vi "getPower.vi"(2 "error in":errorcluster, 3 "AIN Range":u16(ring) items=["LJ_rgBIP10V", "LJ_rgBIP1V", "LJ_rgBIPP1V", "LJ_rgBIPP01V"], 4 "+Channel":u16, 5 "Handle In":i32) -> (0 "error out":errorcluster, 1 "Voltage Reading":dbl)   [LabVIEW 2021]
panel:
  # "inputs"
  # "outputs"
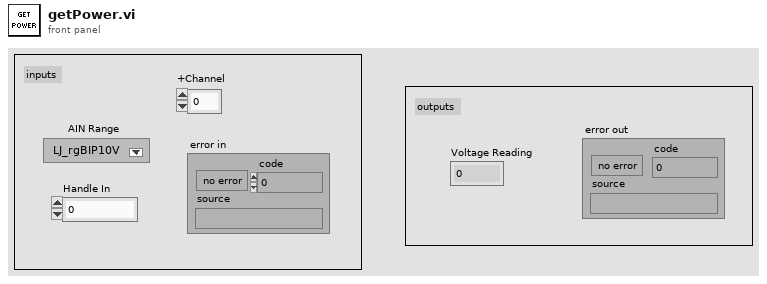
[diagram p1: front panel]
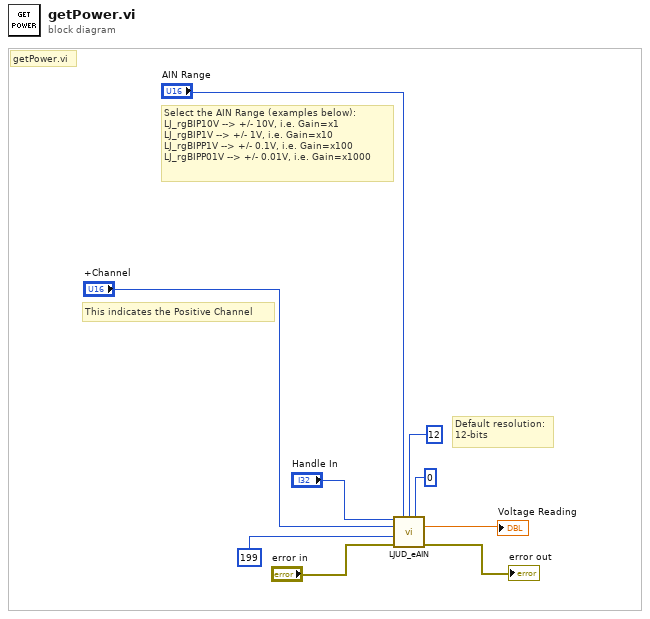
[diagram p0: block diagram]
diagram:
  # "getPower.vi"
  # "This indicates the Positive Channel"
  # "Default resolution:\n12-bits"
  # "Select the AIN Range (examples below):\nLJ_rgBIP10V --> +/- 10V, i.e. Gain=x1\nLJ_rgBIP1V --> +/- 1V, i.e. Gain=x10\nLJ_rgBIPP1V --> +/- 0.1V, i.e. Gain=x100\nLJ_rgBIPP01V --> +/- 0.01V, i.e. Gain=x1000"
  n1 = call <vilib>:"LJUD_eAIN.vi"("Handle In"="Handle In", "Range"="AIN Range", "Resolution"=12, "Settling"=0, "ChannelP"="+Channel", "ChannelN"=199, "error in"="error in") -> ("Voltage"=→"Voltage Reading":dbl, "error out"=→"error out":errorcluster)  [unwired: 6 in, 1 out]
